vi "Write_to_file.vi"() -> ()   [LabVIEW 2022 SP3]
uses:
  <vilib>/sound2/lvsound2.llb/Sound Data Format.ctl
panel:
  in  "path":path
  in  "Tab Control":T1(tab)=enum."STFT Info"
  in  "sound format":T2={"sample rate (S/s)"=44100.0, "number of channels"=1, "bits per sample"=16}
  in  "Duration (s)":dbl=0.1
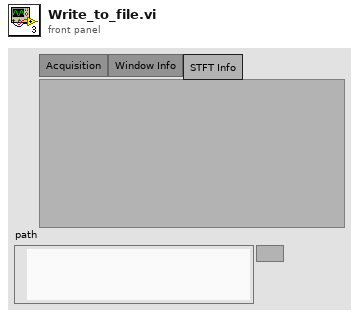
[diagram p1: front panel]
types:
  T1 = enum32{"Acquisition", "Window Info", "STFT Info"}
  T2 = typedef "Sound Data Format.ctl" = cluster{"sample rate (S/s)":dbl, "number of channels":i32, "bits per sample":i32}
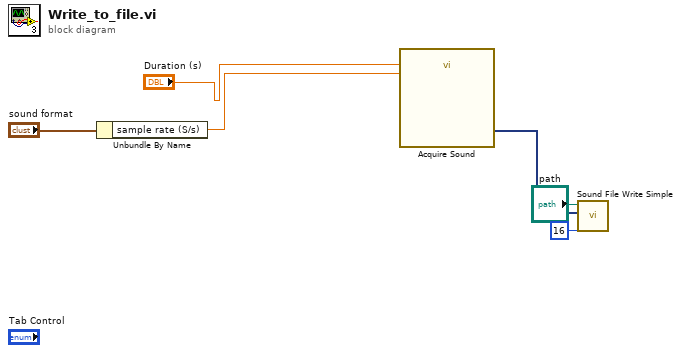
[diagram p0: block diagram]
diagram:
  n1 = Unbundle By Name("sound format") -> ("sample rate (S/s)"=w2:dbl)
  n2 = call "Acquire Sound"("Duration (s)"="Duration (s)", "Sample rate (Hz)"=w2) -> ("Data"=w3:dynamicdata)  [unwired: 16 in, 1 out]
  n3 = call <vilib>:"Sound File Write Simple.vi"("bits per sample"=16, "data"=w3, "path"="path") -> ()  [unwired: 7 in, 2 out]
